vi "Ex2PTGCameras.vi"() -> ()   [LabVIEW 2010]
panel:
  in  "Freq 2":dbl=1000.0 format="%.2f"
  in  "Pulser Gate Width 2":dbl=700.0 format="%.2f"
  in  "Pulser Gate Delay 2":dbl=700.0 format="%.2f"
  in  "On chip accumulation 2":u32=1 min=1 step=1
  in  "Intensifier Gain 2":u32=20
  in  "Gate Mode 2":u32=2 min=1 max=3 step=1
  in  "Temperature 2":dbl=-10.0 format="%.2f"
  in  "Exposure 2":dbl format="%.2f"
  in  "Store 2":bool
  in  "stop 2":bool
  in  "error in (no error)":errorcluster
  in  "Freq":dbl=1000.0 format="%.2f"
  in  "Pulser Gate Width":dbl=700.0 format="%.2f"
  in  "Pulser Gate Delay":dbl=700.0 format="%.2f"
  in  "On chip accumulation":u32=1 min=1 step=1
  in  "Intensifier Gain":u32=20
  in  "Gate Mode":u32=2 min=1 max=3 step=1
  in  "Exposure":dbl format="%.2f"
  in  "Temperature":dbl=-10.0 format="%.2f"
  in  "Store 1":bool
  in  "stop 1":bool
  out "error out":errorcluster
  # "Ex2PTGCameras:\nThis example sets up two PI-Max/PTG\nsystems for internal triggering and \ncollects the images and displays them\nin separate windows. \nRemember to setup the SIPulsers.ini\nThis file should have two entries:\n[PTG1]\n[PTG2]"
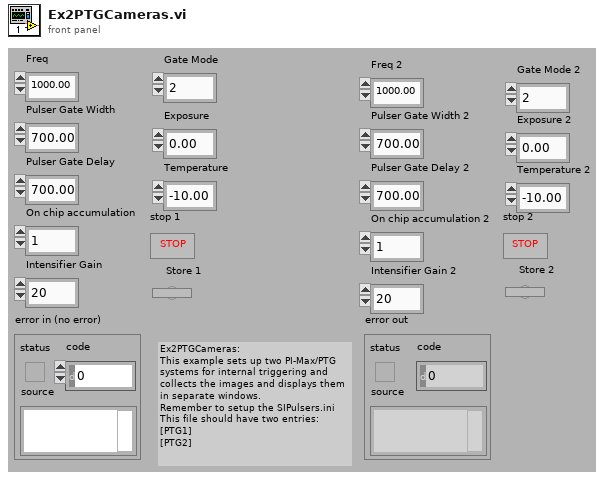
[diagram p1: front panel]
types:
  T1 = cluster{"Freq":dbl, "Pulser Gate Width":dbl, "Pulser Gate Delay":dbl, "On chip accumulation":u32, "Gate Mode":u32, "Intensifier Gain":u32}
  T2 = cluster{"Freq 2":dbl, "Pulser Gate Width 2":dbl, "Pulser Gate Delay 2":dbl, "On chip accumulation 2":u32, "Gate Mode 2":u32, "Intensifier Gain 2":u32}
  T3 = cluster{"Camera Handle":u32, "Pulser Handle":u32, "File Handle":u32, "Display Handle":u32, "Image Handle":u32}
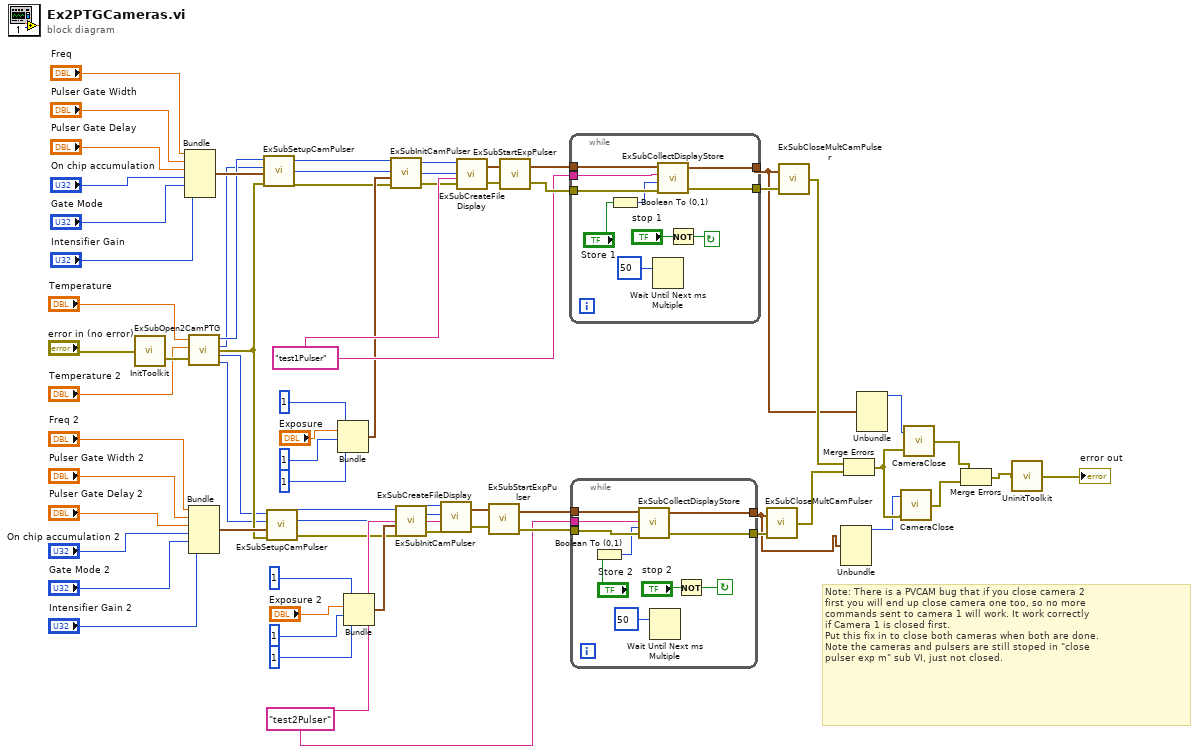
[diagram p0: block diagram]
diagram:
  w38 = "test2Pulser"
  w63 = "test1Pulser"
  # "Note: There is a PVCAM bug that if you close camera 2\nfirst you will end up close camera one too, so no more \ncommands sent to camera 1 will work. It work correctly\nif Camera 1 is closed first. \nPut this fix in to close both cameras when both are done.\nNote the cameras and pulsers are still stoped in \"close\npulser exp m\" sub VI, just not closed."
  n1 = call <userlib>:"InitToolkit.vi"("error in"="error in (no error)") -> ("error out"=w16:errorcluster)
  n2 = Bundle("Freq"="Freq", "Pulser Gate Width"="Pulser Gate Width", "Pulser Gate Delay"="Pulser Gate Delay", "On chip accumulation"="On chip accumulation", "Gate Mode"="Gate Mode", "Intensifier Gain"="Intensifier Gain") -> (w45:T1)  [unwired: 1 in]
  n3 = call "ExSubOpen2CamPTG.vi"("Temperature"="Temperature", "Temperature 2"="Temperature 2", "error in (no error)"=w16) -> ("Camera Handle"=w12:u32, "Pulser Handle"=w11:u32, "Camera Handle 2"=w10:u32, "Pulser Handle 2"=w9:u32, "error out"=w13:errorcluster)
  n4 = Bundle("Freq 2"="Freq 2", "Pulser Gate Width 2"="Pulser Gate Width 2", "Pulser Gate Delay 2"="Pulser Gate Delay 2", "On chip accumulation 2"="On chip accumulation 2", "Gate Mode 2"="Gate Mode 2", "Intensifier Gain 2"="Intensifier Gain 2") -> (w20:T2)  [unwired: 1 in]
  n5 = call "ExSubSetupCamPulser.vi"("error in (no error)"=w13, "Pulser data in"=w45, "Pulser Handle"=w11, "Camera Handle"=w12) -> ("error out"=w48:errorcluster, "Pulser Handle"=w47:u32, "Camera Handle"=w46:u32)
  n6 = call "ExSubSetupCamPulser.vi"("error in (no error)"=w13, "Pulser data in"=w20, "Pulser Handle"=w9, "Camera Handle"=w10) -> ("error out"=w23:errorcluster, "Pulser Handle"=w22:u32, "Camera Handle"=w21:u32)
  n7 = Bundle(1, "Exposure"="Exposure", 1, 1) -> (w55:cluster{i32, "Exposure":dbl, i32, i32})  [unwired: 1 in]
  n8 = Bundle(1, "Exposure 2"="Exposure 2", 1, 1) -> (w30:cluster{i32, "Exposure 2":dbl, i32, i32})  [unwired: 1 in]
  n9 = call "ExSubInitCamPulser.vi"("error in (no error)"=w48, "Camera Information"=w55, "Pulser Handle"=w47, "Camera Handle"=w46) -> ("error out"=w62:errorcluster, "Pulser Handle"=w61:u32, "Camera Handle"=w60:u32)
  n10 = call "ExSubInitCamPulser.vi"("error in (no error)"=w23, "Camera Information"=w30, "Pulser Handle"=w22, "Camera Handle"=w21) -> ("error out"=w37:errorcluster, "Pulser Handle"=w36:u32, "Camera Handle"=w35:u32)
  n11 = call "ExSubCreateFileDisplay.vi"("error in (no error)"=w37, "File and Display Name"=w38, "Pulser Handle"=w36, "Camera Handle"=w35) -> ("error out"=w39:errorcluster, "Handles Out"=w40:T3)
  n12 = call "ExSubCreateFileDisplay.vi"("error in (no error)"=w62, "File and Display Name"=w63, "Pulser Handle"=w61, "Camera Handle"=w60) -> ("error out"=w64:errorcluster, "Handles Out"=w65:T3)
  n13 = call "ExSubStartExpPulser.vi"("error in (no error)"=w39, "Handles In"=w40) -> ("error out"=w41:errorcluster, "Handles Out"=w42:T3)
  n14 = call "ExSubStartExpPulser.vi"("error in (no error)"=w64, "Handles In"=w65) -> ("error out"=w66:errorcluster, "Handles Out"=w67:T3)
  n15 = while {
    tunnel: w67 -> [w78]
    tunnel: w66 -> [w75]
    tunnel: w63 -> [w74]
    tunnel: [w76] -> w68
    tunnel: [w77] -> w5
    stop <- w71 continue-if-true
    n16 = Boolean To (0,1)(Boolean="Store 1") -> (0, 1=w70:i16)
    n17 = Wait Until Next ms Multiple(millisecond multiple=50) -> ()  [unwired: 1 out]
    n18 = call "ExSubCollectDisplayStore.vi"("error in (no error)"=w75, "Store flag"=w70, "Display Title"=w74, "Handle Cluster"=w78) -> ("error out"=w76:errorcluster, "Handle Cluster Out"=w77:T3)  [unwired: 1 out]
    n19 = Not(x="stop 1") -> (.not. x?=w71:bool)
  }
  n20 = while {
    tunnel: w42 -> [w88]
    tunnel: w41 -> [w85]
    tunnel: w38 -> [w84]
    tunnel: [w86] -> w43
    tunnel: [w87] -> w4
    stop <- w81 continue-if-true
    n21 = Boolean To (0,1)(Boolean="Store 2") -> (0, 1=w80:i16)
    n22 = call "ExSubCollectDisplayStore.vi"("error in (no error)"=w85, "Store flag"=w80, "Display Title"=w84, "Handle Cluster"=w88) -> ("error out"=w86:errorcluster, "Handle Cluster Out"=w87:T3)  [unwired: 1 out]
    n23 = Wait Until Next ms Multiple(millisecond multiple=50) -> ()  [unwired: 1 out]
    n24 = Not(x="stop 2") -> (.not. x?=w81:bool)
  }
  n25 = call "ExSubCloseMultCamPulser.vi"("error in (no error)"=w43, "Handles In"=w4) -> ("error out"=w19:errorcluster)
  n26 = call "ExSubCloseMultCamPulser.vi"("error in (no error)"=w68, "Handles In"=w5) -> ("error out"=w18:errorcluster)
  n27 = Unbundle(w4) -> ("Camera Handle"=w3:u32)  [unwired: 4 out]
  n28 = Merge Errors(w18, w19) -> (w8:errorcluster)
  n29 = Unbundle(w5) -> ("Camera Handle"=w2:u32)  [unwired: 4 out]
  n30 = call <userlib>:"CameraClose.vi"("error in"=w8, "Camera Handle"=w3) -> ("error out"=w6:errorcluster)
  n31 = call <userlib>:"CameraClose.vi"("error in"=w8, "Camera Handle"=w2) -> ("error out"=w7:errorcluster)
  n32 = Merge Errors(w7, w6) -> (w1:errorcluster)
  n33 = call <userlib>:"UninitToolkit.vi"("error in"=w1) -> ("error out"=→"error out":errorcluster)
